vi "PTSequencer.ProcEvents.vi"(0 "i ref in":refnum<vi>, 5 "error in":errorcluster) -> (14 "i ref out":refnum<vi>, 19 "error out":errorcluster)   [LabVIEW 2014, in "PTSequencer.lvlib"]
uses:
  PTSequencer.lvlib
  CS_Core/BaseProcess/BaseProcess.event definition.ctl
  CS_Core/CAEObj/CAEObj.event definition.ctl
  CS_Core/BaseProcess/BaseProcess.descriptor string definition.ctl
  CS_Core/BaseProcess/BaseProcess.lvlib
  CS_Core/CAEObj/CAEObj.lvlib
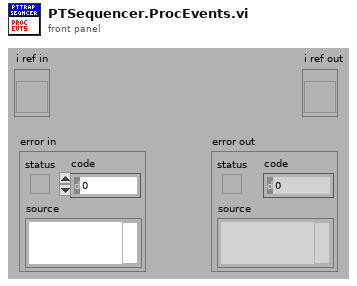
[diagram p1: front panel]
types:
  T1 = typedef "BaseProcess.lvlib/BaseProcess.event definition.ctl" = cluster{"CAEEvtDef":T2, "Data Descriptor":T3}
  T2 = typedef "CAEObj.lvlib/CAEObj.event definition.ctl" = cluster{"URL":string, "enable":bool, "ignoreResID":bool}
  T3 = typedef "BaseProcess.lvlib/BaseProcess.descriptor string definition.ctl" = string
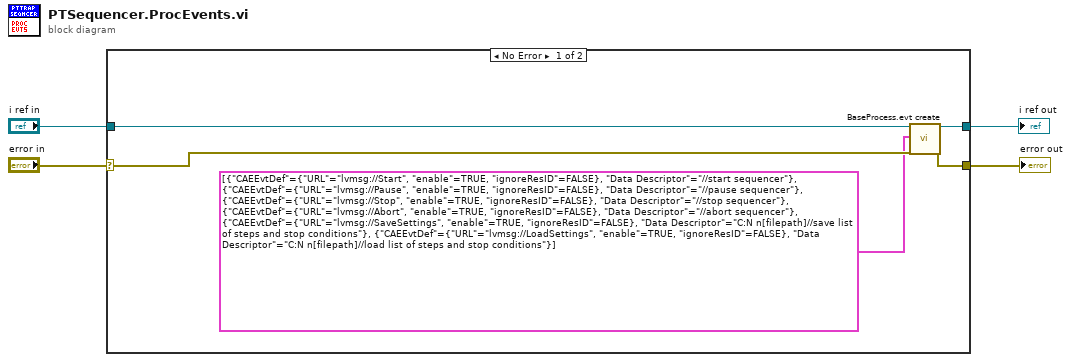
[diagram p0: block diagram]
diagram:
  n1 = case shown="No Error" "error in" {
    selector: "error in" -> [w7 w10]
    tunnel: "i ref in" -> [w6 w11]
    tunnel: [w9 w11] -> w3
    tunnel: [w8 w10] -> w2
    frame No Error {
      n2 = call "BaseProcess.evt create.vi"("i ref in"=w6, "newEvents"=T1[] [{"CAEEvtDef"={"URL"="lvmsg://Start", "enable"=TRUE, "ignoreResID"=FALSE}, "Data Descriptor"="//start sequencer"}, {"CAEEvtDef"={"URL"="lvmsg://Pause", "enable"=TRUE, "ignoreResID"=FALSE}, "Data Descriptor"="//pause sequencer"}, {"CAEEvtDef"={"URL"="lvmsg://Stop", "enable"=TRUE, "ignoreResID"=FALSE}, "Data Descriptor"="//stop sequencer"}, {"CAEEvtDef"={"URL"="lvmsg://Abort", "enable"=TRUE, "ignoreResID"=FALSE}, "Data Descriptor"="//abort sequencer"}, {"CAEEvtDef"={"URL"="lvmsg://SaveSettings", "enable"=TRUE, "ignoreResID"=FALSE}, "Data Descriptor"="C:N n[filepath]//save list of steps and stop conditions"}, {"CAEEvtDef"={"URL"="lvmsg://LoadSettings", "enable"=TRUE, "ignoreResID"=FALSE}, "Data Descriptor"="C:N n[filepath]//load list of steps and stop conditions"}] ("new events"), "error in (no error)"=w7) -> ("i ref out"=w9:refnum<vi>, "error out"=w8:errorcluster)  [unwired: 13 in, 2 out]
    }
    frame Error {
    }
  }
  "i ref out" <- w3
  "error out" <- w2
